vi "myRIO_BRig_Host_stateIdxList_reward.vi"() -> (1 "output_min_reward":u16=32, 3 "output_max_reward":u16=35)   [LabVIEW 2014]
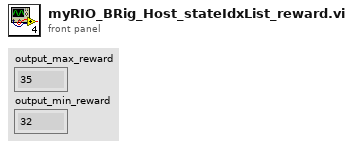
[diagram p1: front panel]
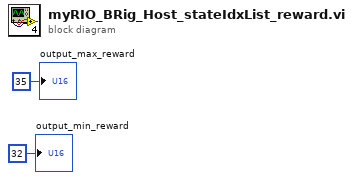
[diagram p0: block diagram]
diagram:
  "output_max_reward" <- u16 35
  "output_min_reward" <- u16 32
